vi "Configure Spectral (Magnitude).vi"(0 "VISA resource name":refnum<visa-resource-name>, 1 "Frequency Span (100kHz)":dbl=100000.0, 2 "Resolution BW (400Hz)":dbl=400000.0, 3 "Gate Position (0s)":dbl, 5 "Channel (4:Math1)":u16(ring)=4 items=["Math1"=4, "Math2"=5, "Math3"=6, "Math4"=7], 7 "Scale (0:Linear)":u16(ring) items=["Linear", "dBm", "dB"], 11 "error in (no error)":errorcluster, 12 "Ref Level (0dB)":dbl, 13 "Ref Level Offset (0V)":dbl, 14 "Window Type (0:Rectangular)":u16(ring) items=["Rectangular", "Hamming", "Hanning", "KaiserBessel", "Black-Harris", "Flattop2", "Gaussian", "TekExp"]) -> (4 "VISA resource name out":refnum<visa-resource-name>, 15 "error out":errorcluster)   [LabVIEW 2015, in "Tektronix 7000 Series.lvlib"]
doc: "Configures the spectral magnitude for a specified mathematical waveform."
uses:
  <instrlib>/Tektronix 7000 Series/Tektronix 7000 Series.lvlib
panel:
  # "Basic Configure"
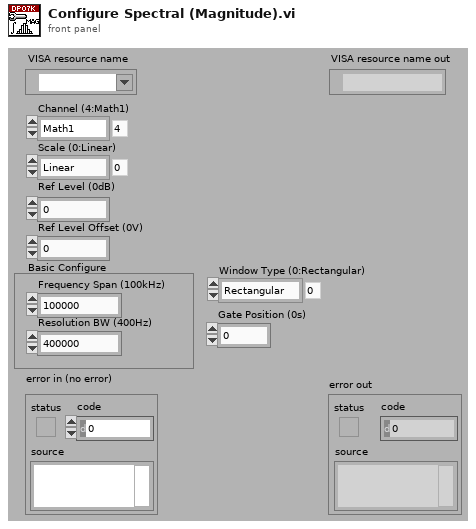
[diagram p1: front panel]
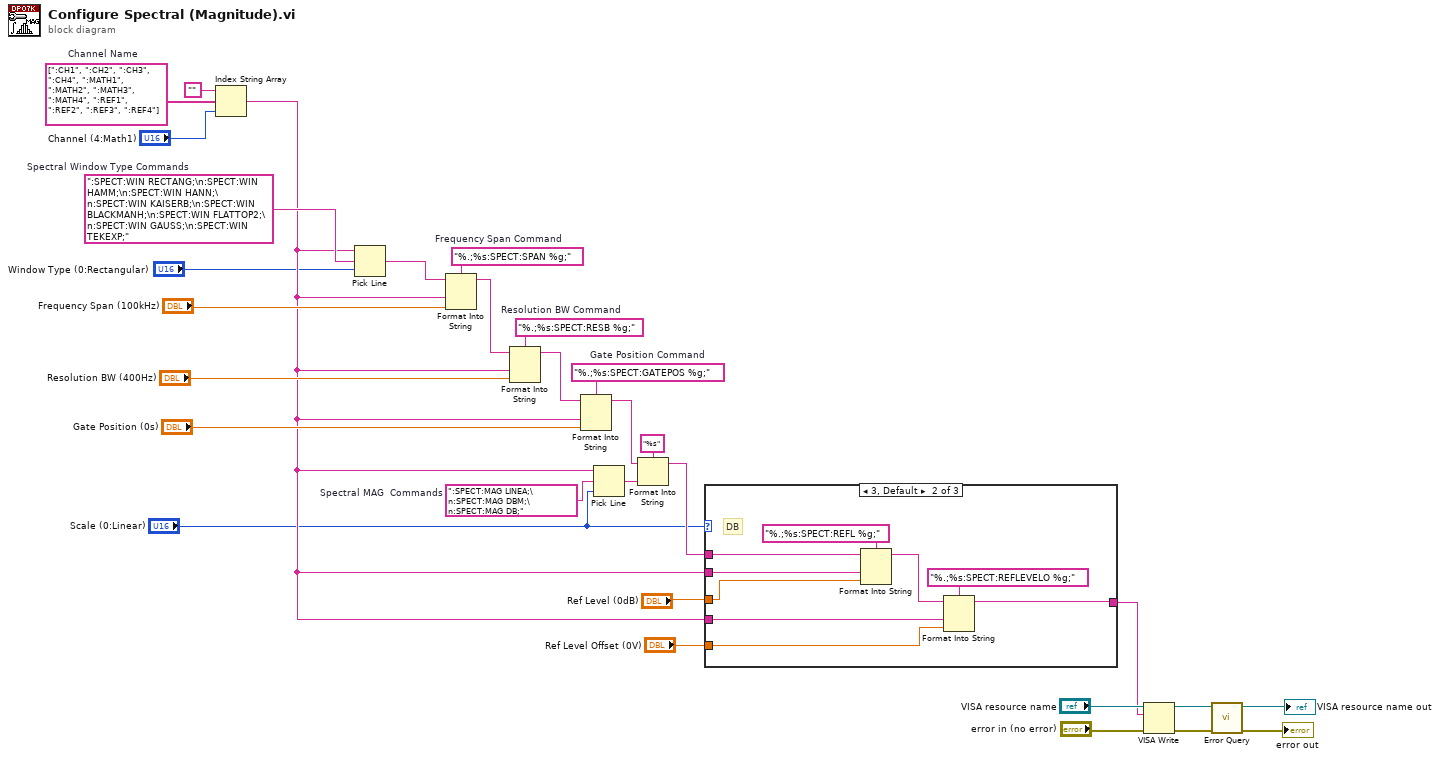
[diagram p0: block diagram]
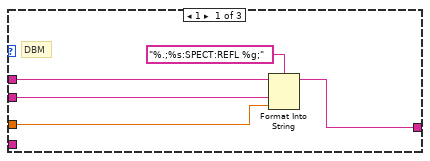
[diagram p2: hidden frame]
diagram:
  w19 = ":SPECT:MAG LINEA;\n:SPECT:MAG DBM;\n:SPECT:MAG DB;"  # Spectral MAG  Commands
  w10 = "%.;%s:SPECT:GATEPOS %g;"  # Gate Position Command
  w22 = ":SPECT:WIN RECTANG;\n:SPECT:WIN HAMM;\n:SPECT:WIN HANN;\n:SPECT:WIN KAISERB;\n:SPECT:WIN BLACKMANH;\n:SPECT:WIN FLATTOP2;\n:SPECT:WIN GAUSS;\n:SPECT:WIN TEKEXP;"  # Spectral Window Type Commands
  w30 = "%.;%s:SPECT:RESB %g;"  # Resolution BW Command
  w28 = "%.;%s:SPECT:SPAN %g;"  # Frequency Span Command
  w27 = string[] [":CH1", ":CH2", ":CH3", ":CH4", ":MATH1", ":MATH2", ":MATH3", ":MATH4", ":REF1", ":REF2", ":REF3", ":REF4"]  # Channel Name
  n1 = Index String Array(1:"Channel (4:Math1)", 2:w27, 3:"" ("Empty String Constant")) -> (0:w7:string)
  n2 = Pick Line(string ("")=w7, multi-line string=w22, line index="Window Type (0:Rectangular)") -> (output string=w6:string)
  n3 = Format Into String(format string=w28, initial string=w6, w7, "Frequency Span (100kHz)") -> (resulting string=w29:string)  [unwired: 1 in, 1 out]
  n4 = Format Into String(format string=w30, initial string=w29, w7, "Resolution BW (400Hz)") -> (resulting string=w5:string)  [unwired: 1 in, 1 out]
  n5 = Format Into String(format string=w10, initial string=w5, w7, "Gate Position (0s)") -> (resulting string=w8:string)  [unwired: 1 in, 1 out]
  n6 = Pick Line(string ("")=w7, multi-line string=w19, line index="Scale (0:Linear)") -> (output string=w21:string)
  n7 = Format Into String(format string="%s", initial string=w8, w21) -> (resulting string=w18:string)  [unwired: 1 in, 1 out]
  n8 = case shown="3, Default" "Scale (0:Linear)" {
    tunnel: w18 -> [w35 w44 w45]
    tunnel: w7 -> [w34 w43 _]
    tunnel: w7 -> [_ w41 _]
    tunnel: [w31 w38 w45] -> w11
    tunnel: "Ref Level Offset (0V)" -> [_ w37 _]
    tunnel: "Ref Level (0dB)" -> [w32 w36 _]
    frame 1 {
      # "DBM"
      n9 = Format Into String(format string="%.;%s:SPECT:REFL %g;", initial string=w35, w34, w32) -> (resulting string=w31:string)  [unwired: 1 in, 1 out]
    }
    frame 3, Default {
      # "DB"
      n10 = Format Into String(format string="%.;%s:SPECT:REFL %g;", initial string=w44, w43, w36) -> (resulting string=w40:string)  [unwired: 1 in, 1 out]
      n11 = Format Into String(format string="%.;%s:SPECT:REFLEVELO %g;", initial string=w40, w41, w37) -> (resulting string=w38:string)  [unwired: 1 in, 1 out]
    }
    frame 0 {
    }
  }
  n12 = VISA Write(VISA resource name="VISA resource name", write buffer=w11, error in (no error)="error in (no error)") -> (VISA resource name out=w17:refnum<visa-resource-name>, error out=w16:errorcluster)  [unwired: 1 out]
  n13 = call <instrlib>:"Error Query.vi"("error in (no error)"=w16, "VISA resource name"=w17) -> ("error out"=→"error out":errorcluster, "VISA resource name out"=→"VISA resource name out":refnum<visa-resource-name>)  [unwired: 6 in, 2 out]
